vi "MoveMultiDrives.vi"(0 "Start Counter":dbl[](array[numeric]), 1 "Matched Configurations In":T2[](array[typedef]) {"Static Drive Configuration"."Indexer Mode  (FSA)" items=["Incremental", "Absolute"]; "Static Drive Configuration"."Buffer at Stop (SSH)" items=["Clear buffer", "Save and Continue"]; "Static Drive Configuration"."Buffer at Limit (SSG)" items=["Clear buffer", "Save and Continue"]; "Static Drive Configuration"."RS232 Echo Control (SSA)" items=["Echo ON", "Echo OFF"]; "Static Drive Configuration"."Reference edge of Home (OSH)" items=["CW", "CCW"]; "Static Drive Configuration"."Encoder Z for Home (OSD)" items=["Don't use", "Enable"]; "Static Drive Configuration"."Home Switch Sense (OSC)" items=["Normally Open", "Normally Closed"]; "Static Drive Configuration"."Home Position (OSB)" items=["Anywhere in Switch", "Edge of Switch"]; "Static Drive Configuration"."Limit Switch Sense (OSA)" items=["Normally Closed", "Normally Open"]; "Static Drive Configuration"."Limit Disable (LD)" items=["Both Enabled", "CW Disabled", "CCW Disabled", "Both Disabled"]; "Static Drive Configuration"."Stall Detect (FSH)" items=["Disable", "Enable"]; "Static Drive Configuration"."OP2 in Deadband (FSG)" items=["Don't Use", "ACTIVATE"]; "Static Drive Configuration"."Stop on Trigger 3 (FSF)" items=["Ignore", "STOP!"]; "Static Drive Configuration"."Activate OP1 on stall (FSE)" items=["Do not Activate", "ACTIVATE!"]; "Static Drive Configuration"."Stop on Stall (FSD)" items=["Continue", "STOP"]; "Static Drive Configuration"."Position Maintenance (FSC)" items=["Disabled", "Enabled"]; "Static Drive Configuration"."Step Mode  (FSB)" items=["Motor", "Encoder"]; "Static Drive Configuration"."Encoder Resolution (ER)" min=1 max=50000; "Static Drive Configuration"."Dead Band Window (DW)" min=0 max=999999999; "Static Drive Configuration"."Dead Band (DB)" min=0 max=999999999; "Static Drive Configuration"."Correction Gain % (CG)" items=["n/a", "12.5", "25", "37.5", "50", "62.5", "75", "87.5", "100"]; "Channel Properties"."Current Pos" format="%.2f"; "Channel Properties"."Backlash/Eng units" format="%.2f"; "Channel Properties"."Pulses/rev" format="%.2f"; "Channel Properties"."Pos Tolerance" format="%.2f"; "Channel Properties"."Pulses/unit" format="%.2f"; "Channel Properties"."Acc. Min" format="%.2f"; "Channel Properties"."Acc. Max" format="%.2f"; "Channel Properties"."Vel. Min" format="%.2f"; "Channel Properties"."Vel. Max" format="%.2f"; "Channel Properties"."Acc. Default" format="%.2f"; "Channel Properties"."Vel. Default" format="%.2f"}, 2 "GoTo Array (pulse position some channels)":T5[](array[typedef]) {"Acceleration" format="%.2f"; "Velocity" format="%.2f"; "Go To Position" step=100000.0}, 3 "Final move":bool, 4 "Predicted Move Time":dbl format="%.2f") -> (5 "Error string":string, 6 "Stop Pressed?":bool, 7 "Matched Configurations Out":T2[](array[typedef]) {"Static Drive Configuration"."Indexer Mode  (FSA)" items=["Incremental", "Absolute"]; "Static Drive Configuration"."Buffer at Stop (SSH)" items=["Clear buffer", "Save and Continue"]; "Static Drive Configuration"."Buffer at Limit (SSG)" items=["Clear buffer", "Save and Continue"]; "Static Drive Configuration"."RS232 Echo Control (SSA)" items=["Echo ON", "Echo OFF"]; "Static Drive Configuration"."Reference edge of Home (OSH)" items=["CW", "CCW"]; "Static Drive Configuration"."Encoder Z for Home (OSD)" items=["Don't use", "Enable"]; "Static Drive Configuration"."Home Switch Sense (OSC)" items=["Normally Open", "Normally Closed"]; "Static Drive Configuration"."Home Position (OSB)" items=["Anywhere in Switch", "Edge of Switch"]; "Static Drive Configuration"."Limit Switch Sense (OSA)" items=["Normally Closed", "Normally Open"]; "Static Drive Configuration"."Limit Disable (LD)" items=["Both Enabled", "CW Disabled", "CCW Disabled", "Both Disabled"]; "Static Drive Configuration"."Stall Detect (FSH)" items=["Disable", "Enable"]; "Static Drive Configuration"."OP2 in Deadband (FSG)" items=["Don't Use", "ACTIVATE"]; "Static Drive Configuration"."Stop on Trigger 3 (FSF)" items=["Ignore", "STOP!"]; "Static Drive Configuration"."Activate OP1 on stall (FSE)" items=["Do not Activate", "ACTIVATE!"]; "Static Drive Configuration"."Stop on Stall (FSD)" items=["Continue", "STOP"]; "Static Drive Configuration"."Position Maintenance (FSC)" items=["Disabled", "Enabled"]; "Static Drive Configuration"."Step Mode  (FSB)" items=["Motor", "Encoder"]; "Static Drive Configuration"."Encoder Resolution (ER)" min=1 max=50000; "Static Drive Configuration"."Dead Band Window (DW)" min=0 max=999999999; "Static Drive Configuration"."Dead Band (DB)" min=0 max=999999999; "Static Drive Configuration"."Correction Gain % (CG)" items=["n/a", "12.5", "25", "37.5", "50", "62.5", "75", "87.5", "100"]; "Channel Properties"."Current Pos" format="%.2f"; "Channel Properties"."Backlash/Eng units" format="%.2f"; "Channel Properties"."Pulses/rev" format="%.2f"; "Channel Properties"."Pos Tolerance" format="%.2f"; "Channel Properties"."Pulses/unit" format="%.2f"; "Channel Properties"."Acc. Min" format="%.2f"; "Channel Properties"."Acc. Max" format="%.2f"; "Channel Properties"."Vel. Min" format="%.2f"; "Channel Properties"."Vel. Max" format="%.2f"; "Channel Properties"."Acc. Default" format="%.2f"; "Channel Properties"."Vel. Default" format="%.2f"})   [LabVIEW 2012]
uses:
  ~subVIs/DriveClusterLower.ctl
  ~subVIs/AxisConfigCluster.ctl
  ~subVIs/DriveProperties.ctl
  ~subVIs/DriveStaticConfig.ctl
  ~subVIs/DriveStatus.ctl
  ~subVIs/GenericDriveCommand.ctl
  ~subVIs/DriveConfigGlobal.vi
  Anemometry/Anemometry Sub Vis/Globals/Trav_pos_global.vi
panel:
  out "Live Position":dbl[](array[numeric]) format="%.2f"
  out "Server copy Location":path
  out "Log File":path
  out "Move Terminated on Timeout":bool
  in  "Axis info cluster":T1
  out "Start Time":dbl format="%.2f"
  out "Running":bool
  out "Bar2":dbl(slide)=2.0 scale=0.0..-50.0
  out "Bar1":dbl(slide)=2.0 scale=-24574.0..-24062.0
  out "Bar0":dbl(slide)=2.0 scale=-101171.2..-101376.0
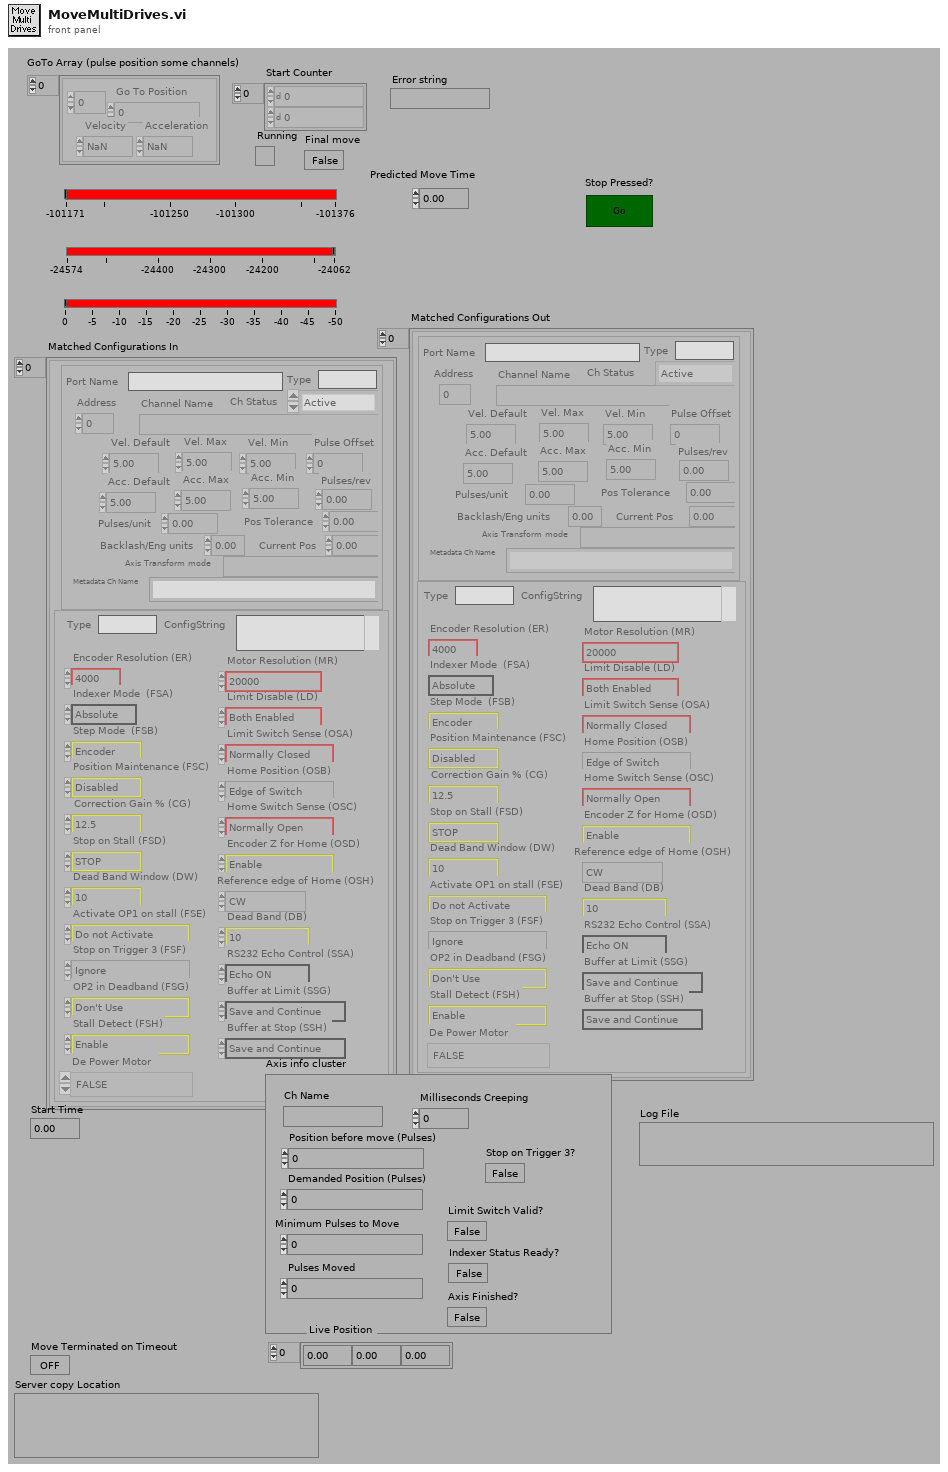
[diagram p1: front panel]
types:
  T1 = typedef "DriveStatus.ctl" = cluster{"Ch Name":string, "Position before move (Pulses)":dbl, "Demanded Position (Pulses)":dbl, "Minimum Pulses to Move":dbl, "Pulses Moved":dbl, "Indexer Status Ready?":bool, "Axis Finished?":bool, "Limit Switch Valid?":bool, "Milliseconds Creeping":u32, "Stop on Trigger 3?":bool}
  T2 = typedef "AxisConfigCluster.ctl" = cluster{"Channel Properties":T3, "Static Drive Configuration":T4}
  T3 = typedef "DriveProperties.ctl" = cluster{"Channel Name":string, "Vel. Default":dbl, "Acc. Default":dbl, "Vel. Max":dbl, "Vel. Min":dbl, "Acc. Max":dbl, "Acc. Min":dbl, "Pulses/unit":dbl, "Address":u8, "Pulse Offset":i32, "Pos Tolerance":dbl, "Pulses/rev":dbl, "Backlash/Eng units":dbl, "Current Pos":dbl, "Ch Status":enum16{"Active", "Offline", "Simulate"}, "Port Name":string, "Axis Transform mode":string, "Metadata Ch Name":string, "Type":string}
  T4 = typedef "DriveStaticConfig.ctl" = cluster{"Correction Gain % (CG)":u16, "Dead Band (DB)":i32, "Dead Band Window (DW)":i32, "Encoder Resolution (ER)":i32, "Step Mode  (FSB)":u16, "Position Maintenance (FSC)":u16, "Stop on Stall (FSD)":u16, "Activate OP1 on stall (FSE)":u16, "Stop on Trigger 3 (FSF)":u16, "OP2 in Deadband (FSG)":u16, "Stall Detect (FSH)":u16, "Limit Disable (LD)":u16, "Motor Resolution (MR)":enum16{"200", "400", "1000", "2000", "4000", "5000", "10000", "12800", "18000", "20000", "21600", "25000", "25400", "25600", "36000", "50000", "278528", "425984", "507904", "614400", "655360", "819200", "1024000"}, "Limit Switch Sense (OSA)":u16, "Home Position (OSB)":u16, "Home Switch Sense (OSC)":u16, "Encoder Z for Home (OSD)":u16, "Reference edge of Home (OSH)":u16, "RS232 Echo Control (SSA)":u16, "Buffer at Limit (SSG)":u16, "Buffer at Stop (SSH)":u16, "Indexer Mode  (FSA)":u16, "Type":string, "ConfigString":string, "De Power Motor":enum16{"TRUE", "FALSE"}}
  T5 = typedef "DriveClusterLower.ctl" = cluster{"Go To Position":dbl, "Velocity":dbl, "Acceleration":dbl, "Address":u8}
  T6 = typedef "GenericDriveCommand.ctl" = string
  T7 = cluster{"GenericDriveCommand":T6, "Go To Position":dbl}
  T8 = cluster{"GenericDriveCommand":T6, "Acceleration":dbl}
  T9 = cluster{"GenericDriveCommand":T6, "Acceleration":dbl}[]
  T10 = enum16{"A-    Acceleration (rps)", "B-    Buffer Status", "C-    Continue", "CG-  Correction Gain", "CR-  Cariage Return", "D-    Distance (pulses)", "DB-  Dead Band (encoder steps)", "DW- Deadband Window (encoder steps)", "E-    Enable Communications", "ER-  Encoder Resolution (steps/rev)", "F-    Disable Communications", "FS-  Encoder Functions Report", "FSA- Incremental/Absolute (0/1)", "FSB- Motor/Encoder Step Mode (0/1)", "FSC- Enable/Disable Position Maint. (1/0)", "FSD- Stop/Continue on Stall (1/0)", "FSE- Activate o/p1 on Stall (1/0)", "FSF- Stop Motion on Trig3 (1/0)", "FSG- Activate o/p2 in Deadband (1/0)", "FSH- Enable Stall Detect (1/0)", "G- Go", "GH- Go Home and Zero (+/-V)", "^H- Delete ", "H- Direction Reverse/CCW/CW (0,1,2)", "IS- Input Status", "K- Kill", "L- Loop (n)", "LD- Limit DISABLE (0-none,1-CW,2-CCW,3-Both)", "LF- Line Feed", "MC- Mode Continuous", "MN- Mode Normal", "MPA- Motor Postion Absolute", "MPI- Motor Position Incremental", "MR- Motor Resolution (Drive Steps/rev)", "N- End of Loop", "O- Output (00,01,10,11)", "OS- Report Homing Setup", "OSA- NO/NC Limits (1/0)", "OSB- Back Up to Home/Edge? (0/1)", "OSC- NO/NC Home Switch (1/0)", "OSD- Enable Encoder Z for Home (0/1)", "OSH- Reference Edge for Home CW/CCW (0/1)", "PR- Report ABSOLUTE Position", "PS- Pause until Continue", "PX- Report Absolute ENCODER Position", "PZ- Zero Absolute Counter", "\"- Quote (17 ASCII +Space)", "Q- Enter/Exit Velocity Profiling (1/0)", "R- Request Indexer Status", "RA- Report Limit Switch Status", "RB- Report Loop, Pause, Shutdown, Trigger Status", "RC- Report Closed Loop Status", "RM- Velocity Streaming Rate Multiplier (000-FFF)", "RV- Report Revision Level", "S- Controlled Stop", "SN- Debounce (1-1000ms)", "SS- Report Software Switch Status", "SSA- Disable RS232 Echo (1/0)", "SSG- Clear/Save Command Buffer on Limit (0/1)", "SSH- Clear/Save Command Buffer on Stop (0/1)", "ST- Shutdown (1/0)", "SV- Servoing Setting (0,1,2,3)", "T- Time Delay (0.01-99999.99)", "TR- Wait for Trigger High/Low/Ignore (1/0/X)", "TS- Report Trigger Status", "U- Pause after Move Until Continue", "V- Velocity (0.01-50.00 revs/sec)", "W1- Report Relative Position <Signed Binary>", "W3- Report Relative Position <Hexadecimal>", "Y- Abort Loop at N", "Z-    Reset to Defaults", "#-    Disable/Set Soft Addresses (0/1-255)"}
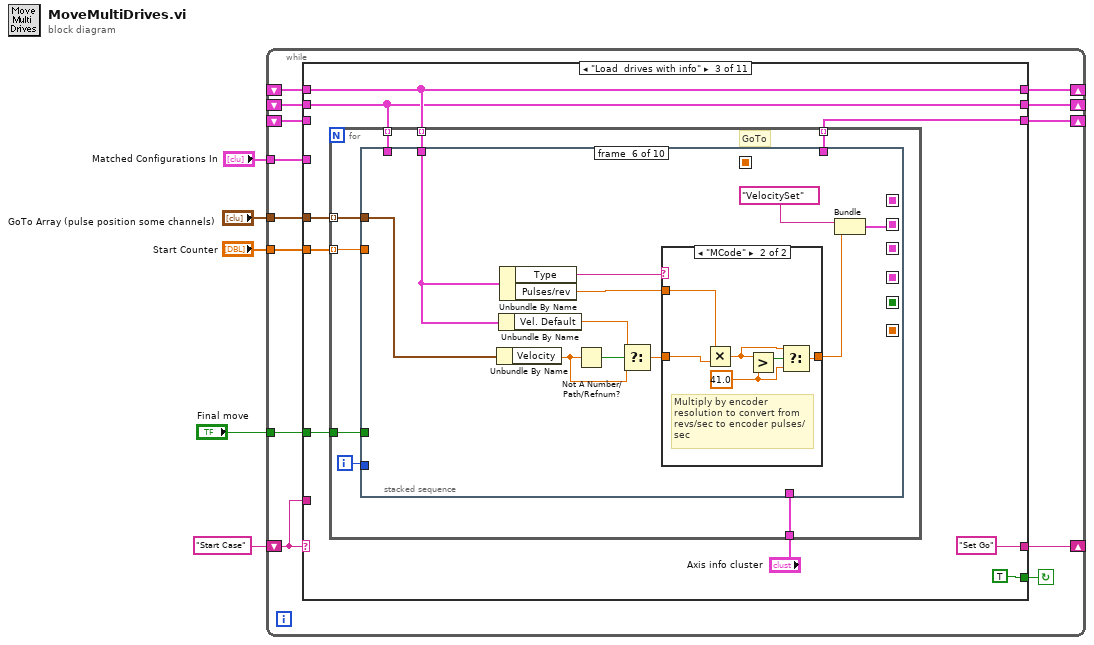
[diagram p0: block diagram]
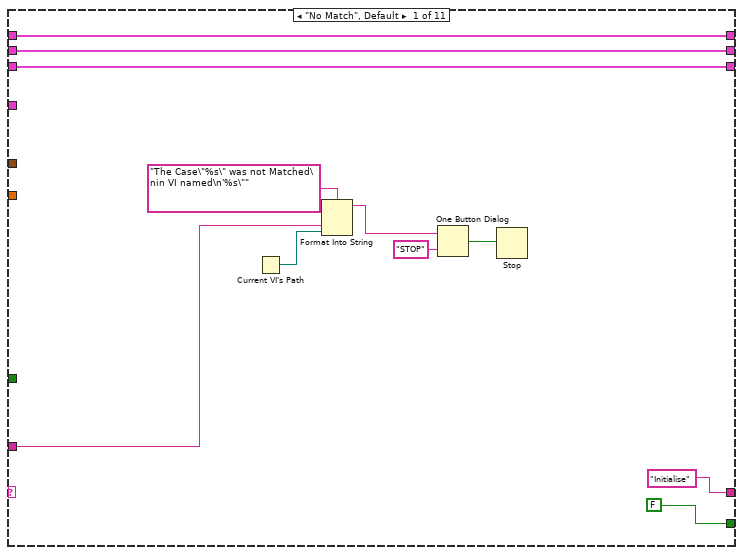
[diagram p2: hidden frame]
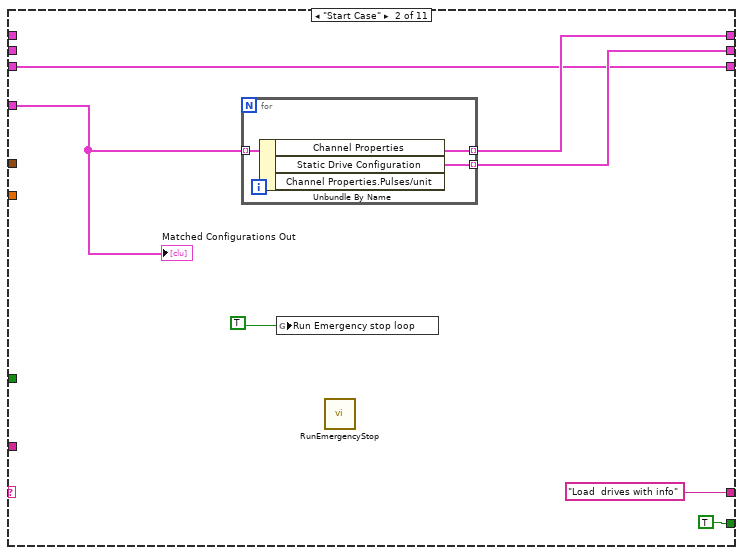
[diagram p3: hidden frame]
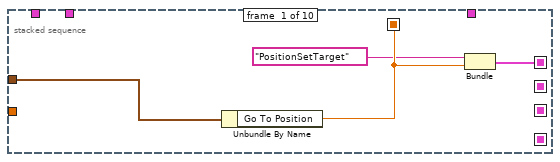
[diagram p4: hidden frame]
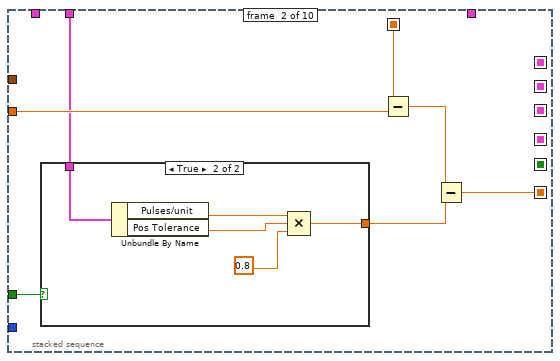
[diagram p5: hidden frame]
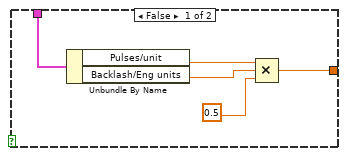
[diagram p6: hidden frame]
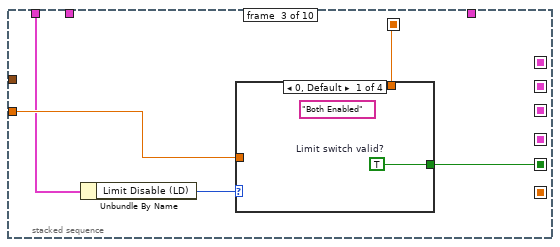
[diagram p7: hidden frame]
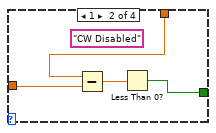
[diagram p8: hidden frame]
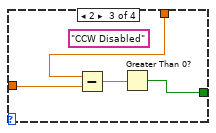
[diagram p9: hidden frame]
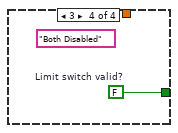
[diagram p10: hidden frame]
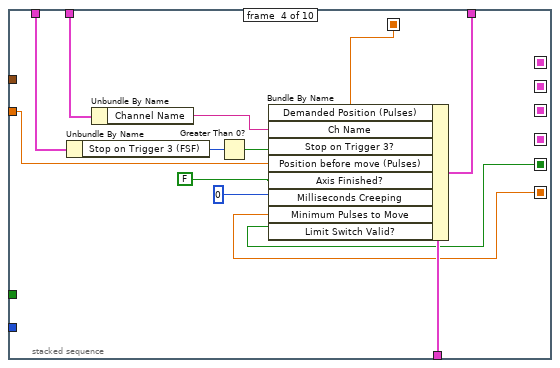
[diagram p11: hidden frame]
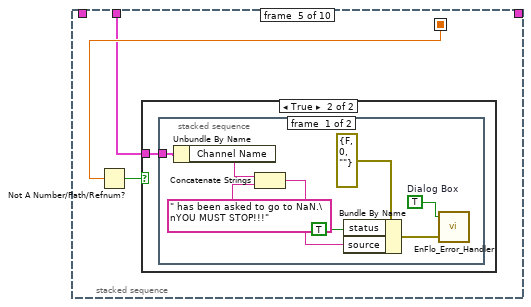
[diagram p12: hidden frame]
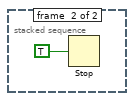
[diagram p14: hidden frame]
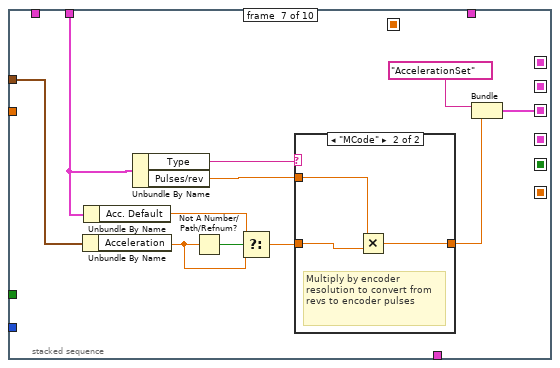
[diagram p16: hidden frame]
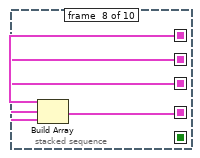
[diagram p18: hidden frame]
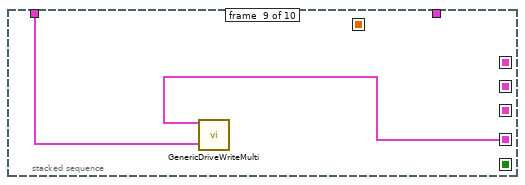
[diagram p19: hidden frame]
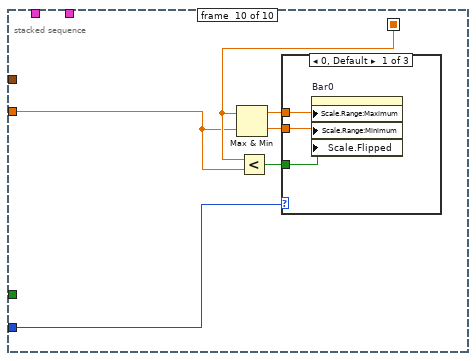
[diagram p20: hidden frame]
diagram:
  n1 = while {
    shift-left: _ -> [w7]
    shift-right: [w6] -> _
    tunnel: "Final move" -> [w8]
    tunnel: "Start Counter" -> [w9]
    tunnel: "GoTo Array (pulse position some channels)" -> [w10]
    tunnel: "Matched Configurations In" -> [w15]
    shift-left: _ -> [w11]
    shift-right: [w13] -> _
    shift-left: _ -> [w12]
    shift-right: [w14] -> _
    shift-left: "Start Case" -> [w16]
    shift-right: [w17] -> _
    stop <- w18 continue-if-true
    n2 = case shown="\"Load  drives with info\"" w16 {
      tunnel: [FALSE TRUE TRUE TRUE TRUE TRUE TRUE TRUE TRUE TRUE FALSE] -> w18
      tunnel: ["Initialise" "Load  drives with info" "Set Go" "Record Time" "Check status of axis" "Continue looping?" w256 "Does Log file Exist" w298 "Write to Log file" "End"] -> w17
      tunnel: w16 -> [w24 _ _ _ _ _ _ _ _ _ _]
      tunnel: w15 -> [_ w30 _ w175 _ _ _ _ _ _ _]
      tunnel: [w21 w33 w45 w179 w190 w197 w275 w287 w303 w324 w351] -> w14
      tunnel: [w20 w32 w42 w178 w189 w198 w274 w286 w302 w323 w350] -> w13
      tunnel: w12 -> [w21 _ w45 w179 w190 w197 w275 w287 w303 w324 w351]
      tunnel: w11 -> [w20 _ w42 w178 w189 w198 w274 w286 w302 w323 w350]
      tunnel: w10 -> [_ _ w46 _ _ _ _ _ _ _ _]
      tunnel: w9 -> [_ _ w44 _ _ _ _ _ _ _ _]
      tunnel: w8 -> [_ _ w43 _ _ _ _ _ _ _ _]
      tunnel: [w19 w31 w40 w176 w187 w193 w261 w285 w301 w322 w348] -> w6
      tunnel: w7 -> [w19 w31 _ w176 w187 w194 w261 w285 w301 w322 w348]
      frame "No Match", Default {
        n3 = Current VI's Path() -> (path=w23:path)
        n4 = Format Into String(format string="The Case\"%s\" was not Matched\nin VI named\n'%s\"" ("Format String"), w24, w23) -> (resulting string=w27:string)  [unwired: 2 in, 1 out]
        n5 = One Button Dialog(message=w27, button name ("OK")="STOP") -> (true=w25:bool)
        n6 = Stop(stop? (T)=w25) -> ()
      }
      frame "Start Case" {
        n7 = for {
          tunnel: w30 -> [w39] mode=indexing
          tunnel: [w38] -> w33 mode=indexing
          tunnel: [w37] -> w32 mode=indexing
          n8 = Unbundle By Name(w39) -> ("Channel Properties"=w38:T3, "Static Drive Configuration"=w37:T4)  [unwired: 1 out]
        }
        n9 = global write "DriveConfigGlobal.vi" "Run Emergency stop loop"(TRUE) -> ()
        n10 = call "RunEmergencyStop.vi"() -> ()  [unwired: 1 in, 7 out]
        "Matched Configurations Out" <- w30
      }
      frame "Load  drives with info" {
        n11 = for {
          tunnel: w46 -> [w55] mode=indexing
          tunnel: w45 -> [w54] mode=indexing
          tunnel: w44 -> [w53] mode=indexing
          tunnel: w43 -> [w52]
          tunnel: w42 -> [w51] mode=indexing
          tunnel: "Axis info cluster" -> [w50]
          tunnel: [w49] -> w40 mode=indexing
          i -> [w56]
          # "GoTo"
          n12 = stacked-sequence {
            seq-local: [w59 _ _ _ _ _ _ _ _ _] -> [_ w67 w81 w96 w108 _ _ _ _ w161]
            seq-local: [w58 _ _ _ _ _ _ _ _ _] -> [_ _ _ _ _ _ _ w155 _ _]
            seq-local: [_ _ _ _ _ w125 _ _ _ _] -> [_ _ _ _ _ _ _ w154 _ _]
            seq-local: [_ _ _ _ _ _ w143 _ _ _] -> [_ _ _ _ _ _ _ w153 _ _]
            seq-local: [_ _ _ _ _ _ _ w152 _ _] -> [_ _ _ _ _ _ _ _ w157 _]
            seq-local: [_ w62 _ _ _ _ _ _ _ _] -> [_ _ _ w103 _ _ _ _ _ _]
            seq-local: [_ _ w78 _ _ _ _ _ _ _] -> [_ _ _ w101 _ _ _ _ _ _]
            tunnel: w55 -> [w60 _ _ _ _ w129 w147 _ _ _]
            tunnel: w56 -> [_ _ _ _ _ _ _ _ _ w158]
            tunnel: w52 -> [_ w65 _ _ _ _ _ _ _ _]
            tunnel: w54 -> [_ w63 _ w105 w106 w123 w141 _ w156 _]
            tunnel: w53 -> [_ w64 w80 w98 _ _ _ _ _ w159]
            tunnel: w51 -> [_ _ w79 w100 _ _ _ _ _ _]
            tunnel: w50 -> [_ _ _ w104 _ _ _ _ _ _]
            tunnel: [_ _ _ w102 _ _ _ _ _ _] -> w49
            frame #0 {
              n13 = Unbundle By Name(w60) -> ("Go To Position"=w59:dbl)
              n14 = Bundle("GenericDriveCommand"=T6 "PositionSetTarget", "Go To Position"=w59) -> (w58:T7)  [unwired: 1 out]
            }
            frame #1 {
              n15 = case shown="True" w65 {
                tunnel: w63 -> [w72 w77]
                tunnel: [w68 w73] -> w66
                frame False {
                  n16 = Unbundle By Name(w72) -> ("Pulses/unit"=w71:dbl, "Backlash/Eng units"=w70:dbl)
                  n17 = Compound Arithmetic op=MULTIPLY(w71, w70, 0.5) -> (w68:dbl)
                }
                frame True {
                  n18 = Unbundle By Name(w77) -> ("Pulses/unit"=w76:dbl, "Pos Tolerance"=w75:dbl)
                  n19 = Compound Arithmetic op=MULTIPLY(w76, w75, 0.8) -> (w73:dbl)
                }
              }
              n20 = Subtract(x=w67, y=w64) -> (x-y=w61:dbl)
              n21 = Subtract(x=w61, y=w66) -> (x-y=w62:dbl)
            }
            frame #2 {
              n22 = Unbundle By Name(w79) -> ("Limit Disable (LD)"=w82:u16)
              n23 = case shown="0, Default" w82 {
                tunnel: [w83 w84 w88 w92] -> w78
                tunnel: w80 -> [_ w86 w90 _]
                tunnel: w81 -> [_ w87 w91 _]
                frame 0, Default {
                  w83 = TRUE  # Limit switch valid?
                  (unwired) "Both Enabled"
                }
                frame 1 {
                  (unwired) "CW Disabled"
                  n24 = Subtract(x=w87, y=w86) -> (x-y=w85:dbl)
                  n25 = Less Than 0?(x=w85) -> (x < 0?=w84:bool)
                }
                frame 2 {
                  (unwired) "CCW Disabled"
                  n26 = Subtract(x=w91, y=w90) -> (x-y=w89:dbl)
                  n27 = Greater Than 0?(x=w89) -> (x > 0?=w88:bool)
                }
                frame 3 {
                  (unwired) "Both Disabled"
                  w92 = FALSE  # Limit switch valid?
                }
              }
            }
            frame #3 {
              n28 = Unbundle By Name(w100) -> ("Stop on Trigger 3 (FSF)"=w99:u16)
              n29 = Unbundle By Name(w105) -> ("Channel Name"=w97:string)
              n30 = Greater Than 0?(x=w99) -> (x > 0?=w95:bool)
              n31 = Bundle By Name(cluster=w104, "Demanded Position (Pulses)"=w96, "Ch Name"=w97, "Stop on Trigger 3?"=w95, "Position before move (Pulses)"=w98, "Axis Finished?"=FALSE ("Bundle Element"), "Milliseconds Creeping"=u32 0 ("Bundle Element"), "Minimum Pulses to Move"=w103, "Limit Switch Valid?"=w101) -> (w102:T1)
            }
            frame #4 {
              n32 = Not A Number/Path/Refnum?(number/path/refnum=w108) -> (NaN/Path/Refnum?=w107:bool)
              n33 = case shown="True" w107 {
                tunnel: w106 -> [_ w109]
                frame False {
                }
                frame True {
                  n34 = stacked-sequence {
                    tunnel: w109 -> [w117 _]
                    frame #0 {
                      w110 = TRUE  # Dialog Box
                      n35 = Unbundle By Name(w117) -> ("Channel Name"=w113:string)
                      n36 = Concatenate Strings(w113, " has been asked to go to NaN.\nYOU MUST STOP!!!") -> (w111:string)
                      n37 = Bundle By Name(cluster=errorcluster {"status"=FALSE, "code"=0, "source"=""} ("error in (no error)"), "status"=TRUE ("Bundle Element"), "source"=w111) -> (w115:errorcluster)
                      n38 = call "EnFlo_Error_Handler.vi"("error in (no error)"=w115, "Dialog Box (T)"=w110) -> ()  [unwired: 1 in, 3 out]
                    }
                    frame #1 {
                      n39 = Stop(stop? (T)=TRUE) -> ()
                    }
                  }
                }
              }
            }
            frame #5 {
              n40 = Unbundle By Name(w129) -> ("Velocity"=w126:dbl)
              n41 = Unbundle By Name(w123) -> ("Vel. Default"=w127:dbl)
              n42 = Unbundle By Name(w123) -> ("Type"=w122:string, "Pulses/rev"=w120:dbl)
              n43 = Not A Number/Path/Refnum?(number/path/refnum=w126) -> (NaN/Path/Refnum?=w128:bool)
              n44 = Select(t=w127, s=w128, f=w126) -> (s? t:f=w121:dbl)
              n45 = case shown="\"MCode\"" w122 {
                tunnel: w121 -> [w130 w131]
                tunnel: w120 -> [_ w136]
                tunnel: [w130 w135] -> w119
                frame "ParkerX", Default {
                }
                frame "MCode" {
                  w132 = 41.0 ("y")
                  # "Multiply by encoder resolution to convert from revs/sec to encoder pulses/sec"
                  n46 = Multiply(x=w136, y=w131) -> (x*y=w133:dbl)
                  n47 = Greater?(x=w133, y=w132) -> (0:w134:bool)
                  n48 = Select(t=w133, s=w134, f=w132) -> (s? t:f=w135:dbl)
                }
              }
              n49 = Bundle("GenericDriveCommand"=T6 "VelocitySet", "y"=w119) -> (w125:cluster{"GenericDriveCommand":T6, "y":dbl})  [unwired: 1 out]
            }
            frame #6 {
              n50 = Unbundle By Name(w147) -> ("Acceleration"=w144:dbl)
              n51 = Unbundle By Name(w141) -> ("Acc. Default"=w145:dbl)
              n52 = Unbundle By Name(w141) -> ("Type"=w140:string, "Pulses/rev"=w139:dbl)
              n53 = Not A Number/Path/Refnum?(number/path/refnum=w144) -> (NaN/Path/Refnum?=w146:bool)
              n54 = Select(t=w145, s=w146, f=w144) -> (s? t:f=w138:dbl)
              n55 = case shown="\"MCode\"" w140 {
                tunnel: w138 -> [w148 w151]
                tunnel: w139 -> [_ w150]
                tunnel: [w148 w149] -> w137
                frame "ParkerX", Default {
                }
                frame "MCode" {
                  # "Multiply by encoder resolution to convert from revs to encoder pulses"
                  n56 = Multiply(x=w150, y=w151) -> (x*y=w149:dbl)
                }
              }
              n57 = Bundle("GenericDriveCommand"=T6 "AccelerationSet", "Acceleration"=w137) -> (w143:T8)  [unwired: 1 out]
            }
            frame #7 {
              n58 = Build Array(w155, w154, w153) -> (w152:T9)
            }
            frame #8 {
              n59 = call "GenericDriveWriteMulti.vi"("Channel Description"=w156, "Array Constant"=w157) -> ()  [unwired: 1 out]
            }
            frame #9 {
              n60 = Max & Min(x=w161, y=w159) -> (max(x,y)=w163:dbl, min(x,y)=w162:dbl)
              n61 = Less?(x=w161, y=w159) -> (x < y?=w160:bool)
              n62 = case shown="0, Default" w158 {
                tunnel: w163 -> [w166 w169 w172]
                tunnel: w162 -> [w165 w168 w171]
                tunnel: w160 -> [w164 w167 w170]
                frame 0, Default {
                  n63 = property on="Bar0" class="Slide (strict)"("Scale.Range:Maximum"=w166, "Scale.Range:Minimum"=w165, "Scale.Flipped"=w164) -> ()  [unwired: 2 in, 2 out]
                }
                frame 1 {
                  n64 = property on="Bar1" class="Slide (strict)"("Scale.Range:Maximum"=w169, "Scale.Range:Minimum"=w168, "Scale.Flipped"=w167) -> ()  [unwired: 2 in, 2 out]
                }
                frame 2 {
                  n65 = property on="Bar2" class="Slide (strict)"("Scale.Range:Maximum"=w172, "Scale.Range:Minimum"=w171, "Scale.Flipped"=w170) -> ()  [unwired: 2 in, 2 out]
                }
              }
            }
          }
        }
      }
      frame "Set Go" {
        n66 = call "GetActivePortNames.vi"("Matched Configurations In"=w175) -> ("Port Name Array"=w174:string[], "Drive Type Array"=w173:string[])
        n67 = for {
          tunnel: w174 -> [w185] mode=indexing
          tunnel: "Global" -> [w184]
          tunnel: w173 -> [w183] mode=indexing
          n68 = call "GenericDriveIO.vi"("GenericDriveCommand"=T6 "GoNow", "Channel Name"=w184, "Type"=w183, "Port Name"=w185) -> ()  [unwired: 2 in, 6 out]
        }
      }
      frame "Record Time" {
        n69 = Get Date/Time In Seconds() -> (seconds since 1Jan1904=w186:timestamp)
        n70 = To Double Precision Float(number=w186) -> (double precision float=→"Start Time":dbl)
      }
      frame "Check status of axis" {
        (unwired) "Global"
        n71 = for {
          shift-right: [w205] -> w195
          shift-left: "" -> [w207]
          tunnel: w197 -> [w206] mode=indexing
          tunnel: w194 -> [w202] mode=indexing
          tunnel: [w201] -> w193 mode=indexing
          i -> [w208]
          n72 = Unbundle By Name(w202) -> ("Axis Finished?"=w203:bool, "Position before move (Pulses)"=w204:dbl)
          n73 = case shown="False" w203 {
            tunnel: w208 -> [w232 _]
            tunnel: w207 -> [w231 w252]
            tunnel: w206 -> [w224 _]
            tunnel: [w229 w252] -> w205
            tunnel: w204 -> [w228 _]
            tunnel: w202 -> [w227 w251]
            tunnel: [w225 w251] -> w201
            frame False {
              n74 = Unbundle By Name(w224) -> ("Channel Name"=w218:string, "Pulses/unit"=w223:dbl, "Pulse Offset"=w220:i32)
              n75 = call "CheckDriveStatus.vi"("Channel Properties"=w224, "Axis info cluster"=w227) -> ("Error string"=w230:string, "Axis info cluster Out"=w225:T1)
              n76 = Unbundle By Name(w225) -> ("Pulses Moved"=w219:dbl)
              n77 = global read "Trav_pos_global.vi" "Live Position"() -> (w210:dbl[])
              n78 = Match Pattern(string=w218, regular expression=":") -> (before substring=w214:string, after substring=w213:string)  [unwired: 1 in, 2 out]
              n79 = Match Pattern(string=w213, regular expression=":") -> (after substring=w212:string)  [unwired: 1 in, 3 out]
              n80 = Add(x=w220, y=w219) -> (x+y=w221:dbl)
              n81 = Divide(x=w221, y=w223) -> (x/y=w211:dbl)
              n82 = case shown="\"Y\"" w212 {
                tunnel: w211 -> [w234 w239 w247]
                tunnel: w210 -> [w236 w242 w246]
                tunnel: [w233 w238 w243] -> w209
                frame "Y" {
                  n83 = Index Array(array=w236) -> (element #1=w235:dbl, element #3=w237:dbl)  [unwired: 3 in, 1 out]
                  n84 = Build Array(w235, w234, w237) -> (w233:dbl[])
                }
                frame "X" {
                  n85 = Index Array(array=w242) -> (element #2=w240:dbl, element #3=w241:dbl)  [unwired: 3 in, 1 out]
                  n86 = Build Array(w239, w240, w241) -> (w238:dbl[])
                }
                frame "Z", Default {
                  n87 = Index Array(array=w246) -> (element #1=w245:dbl, element #2=w244:dbl)  [unwired: 2 in]
                  n88 = Build Array(w245, w244, w247) -> (w243:dbl[])
                }
              }
              n89 = Add(x=w228, y=w219) -> (x+y=w226:dbl)
              n90 = call "Coordinate_transforms.vi"("Traverse Name"=w214, "Input"=w209, "Mode"=enum16{"XYZ to Channel", "Channel to XYZ"}."Channel to XYZ") -> ("Output"=w216:dbl[])
              "Live Position" <- w216
              n91 = Concatenate Strings(w231, w230) -> (w229:string)
              n92 = case shown="2" w232 {
                tunnel: w226 -> [w248 w249 w250]
                frame 0, Default {
                  "Bar0" <- w248
                }
                frame 1 {
                  "Bar1" <- w249
                }
                frame 2 {
                  "Bar2" <- w250
                }
              }
              n93 = global write "Trav_pos_global.vi" "Live Position"(w216) -> ()
            }
            frame True {
            }
          }
        }
        "Error string" <- w195
      }
      frame "Continue looping?" {
        n94 = for {
          tunnel: w261 -> [w278] mode=indexing
          tunnel: [w277] -> w260 mode=indexing
          n95 = Unbundle By Name(w278) -> ("Axis Finished?"=w277:bool)
        }
        n96 = Multiply(x="Predicted Move Time", y=1.1) -> (x*y=w267:dbl)
        n97 = global read "DriveConfigGlobal.vi" "Stop Pressed?"() -> (w270:bool)
        "Stop Pressed?" <- w270
        n98 = Add(x=w267, y=10.0) -> (x+y=w263:dbl)
        n99 = local read "Start Time"() -> (w262:dbl)
        n100 = Get Date/Time In Seconds() -> (seconds since 1Jan1904=w253:timestamp)
        n101 = To Double Precision Float(number=w253) -> (double precision float=w268:dbl)
        n102 = Subtract(x=w268, y=w262) -> (x-y=w269:dbl)
        n103 = local read "Error string"() -> (w271:string)
        n104 = Less?(x=w269, y=w263) -> (x < y?=w255:bool)
        n105 = And Array Elements(Boolean array=w260) -> (logical AND=w273:bool)
        n106 = Not(x=w255) -> (.not. x?=→"Move Terminated on Timeout":bool)
        n107 = Empty String/Path?(string/path=w271) -> (empty?=w272:bool)
        n108 = Compound Arithmetic op=AND(w272, invert w273, invert w270, w255) -> (w259:bool)
        n109 = call "Program_Active.vi"() -> ()  [unwired: 1 in]
        n110 = Select(t="Check status of axis", s=w259, f="Kill All Axes") -> (s? t:f=w256:string)
      }
      frame "Kill All Axes" {
        # "Kill All Axis in case they are creeping"
        n111 = global read "DriveConfigGlobal.vi" "Configurations"() -> (w284:T2[])
        n112 = call "GetActivePortNames.vi"("Matched Configurations In"=w284) -> ("Port Name Array"=w281:string[], "Drive Type Array"=w279:string[])
        n113 = for {
          tunnel: w281 -> [w292] mode=indexing
          tunnel: "Global" -> [w291]
          tunnel: w279 -> [w290] mode=indexing
          (unwired) T10."K- Kill" ("COMMAND")
          n114 = call "GenericDriveIO.vi"("GenericDriveCommand"=T6 "StopEmergency", "Channel Name"=w291, "Type"=w290, "Port Name"=w292) -> ()  [unwired: 2 in, 6 out]
        }
        "Running" <- FALSE
      }
      frame "Does Log file Exist" {
        n115 = call "Create_Error_log_folders.vi"("Per Day Log File?"=TRUE, "Log Filename"="Traverse_Low" ("Input Element")) -> ("exists?"=w295:bool, "Server copy Location"=→"Server copy Location":path, "Local Log File"=→"Log File":path)  [unwired: 1 in]
        n116 = Select(t="Write to Log file", s=w295, f="Create Log file") -> (s? t:f=w298:string)
      }
      frame "Create Log file" {
        n117 = Build Array("Date::", "Time::", "Seconds:Since:1st Jan 1904", "Move:Duration:Seconds", "Move:Terminated:On Timeout") -> (w313:string[])
        n118 = for {
          N: 3 -> [_]
          shift-right: [w326] -> w312
          shift-left: w313 -> [w327]
          i -> [w332]
          n119 = Increment(x=w332) -> (x+1=w331:i32)
          n120 = Number To Decimal String(number=w331) -> (decimal integer string=w330:string)  [unwired: 1 out]
          n121 = Build Array("Axis:Ch Name:", "Position Before:Move (Pulses):", "Demanded:Position (Pulses):", "Minimum Pulses:to Move:", "Pulses:Moved:", "Indexer:Status Ready:", "Axis:Finished?", "Limit:Switch Valid?") -> (w329:string[])
          n122 = for {
            tunnel: w330 -> [w343]
            tunnel: w329 -> [w342] mode=indexing
            tunnel: [w341] -> w328 mode=indexing
            n123 = Concatenate Strings(w342, w343) -> (w341:string)
          }
          n124 = Build Array (concatenate)(w327, w328) -> (w326:string[])
        }
        n125 = for {
          tunnel: w312 -> [w347] mode=indexing
          tunnel: [w346] -> w316 mode=indexing
          tunnel: [w345] -> w317 mode=indexing
          tunnel: [w344] -> w318 mode=indexing
          n126 = call "Split_Ch_name.vi"("Ch name"=w347) -> ("Top level"=w346:string, "Middle"=w345:string, "Low level"=w344:string)
        }
        n127 = local read "Log File"() -> (w305:path)
        n128 = Build Array(w316, w317, w318) -> (w314:string[][])
        n129 = Array To Spreadsheet String(array=w314, 3:"%s" ("format string")) -> (spreadsheet string=w306:string)  [unwired: 1 out]
        n130 = call "Write_File_Simple.vi"("append to file? (new file:F)"=TRUE, "character string"=w306, "file path"=w305) -> ()  [unwired: 2 out]
      }
      frame "Write to Log file" {
        n131 = stacked-sequence {
          seq-local: [w357 _ _] -> [_ w369 _]
          seq-local: [_ w368 _] -> [_ _ w395]
          tunnel: w348 -> [_ w370 _]
          frame #0 {
            n132 = local read "Move Terminated on Timeout"() -> (w364:bool)
            n133 = Get Date/Time In Seconds() -> (seconds since 1Jan1904=w356:timestamp)
            n134 = local read "Start Time"() -> (w366:dbl)
            n135 = To Double Precision Float(number=w356) -> (double precision float=w355:dbl)
            n136 = Subtract(x=w355, y=w366) -> (x-y=w365:dbl)
            n137 = Get Date/Time String(date format (0)=enum16{"short", "long", "abbreviated"}."abbreviated", seconds (now)=w356) -> (date string=w361:string, time string=w360:string)  [unwired: 1 out]
            n138 = Number To Fractional String(number=w355, precision (6)=i16 3) -> (F-format string=w353:string)  [unwired: 2 out]
            n139 = Number To Decimal String(number=w365) -> (decimal integer string=w359:string)  [unwired: 1 out]
            n140 = Select(t="TRUE", s=w364, f="FALSE") -> (s? t:f=w358:string)
            n141 = Build Array(w361, w360, w353, w359, w358) -> (w357:string[])
          }
          frame #1 {
            n142 = for {
              tunnel: w370 -> [w385] mode=indexing
              shift-right: [w373] -> w368
              shift-left: w369 -> [w374]
              n143 = Unbundle By Name(w385) -> ("Ch Name"=w377:string, "Position before move (Pulses)"=w384:dbl, "Demanded Position (Pulses)"=w383:dbl, "Minimum Pulses to Move"=w371:dbl, "Pulses Moved"=w382:dbl, "Indexer Status Ready?"=w381:bool, "Axis Finished?"=w380:bool, "Limit Switch Valid?"=w372:bool)
              n144 = Build Array(w384, w383, w371, w382) -> (w378:dbl[])
              n145 = Build Array(w381, w380, w372) -> (w379:bool[])
              n146 = Number To Decimal String(number=w378) -> (decimal integer string=w376:string[])  [unwired: 1 out]
              n147 = for {
                tunnel: w379 -> [w387] mode=indexing
                tunnel: [w386] -> w375 mode=indexing
                n148 = Select(t="TRUE", s=w387, f="FALSE") -> (s? t:f=w386:string)
              }
              n149 = Build Array (concatenate)(w374, w377, w376, w375) -> (w373:string[])
            }
          }
          frame #2 {
            n150 = for {
              shift-right: [w399] -> w392
              shift-left: "\r\n" -> [w400]
              tunnel: w395 -> [w398] mode=indexing
              n151 = Concatenate Strings(w400, w398, "\t") -> (w399:string)
            }
            n152 = local read "Log File"() -> (w393:path)
            n153 = local read "Server copy Location"() -> (w391:path)
            n154 = call "Write_File_Simple.vi"("append to file? (new file:F)"=TRUE, "character string"=w392, "file path"=w393) -> ("file path Out"=w390:path)  [unwired: 1 out]
            n155 = call "Updated_File_Copy.vi"("Target Path"=w391, "Source Path"=w390) -> ()  [unwired: 2 out]
          }
        }
      }
    }
  }
